vi "holonomic-drive-test.vi"(8 "error in (no error)":errorcluster) -> (0 "error out":errorcluster, 3 "ALL TESTS PASSED":bool)   [LabVIEW 2019]
uses:
  <vilib>/Rock Robotics/WPI/ThirdParty/JAS_Junk/TrajLib/POSE2D.ctl
  <vilib>/Rock Robotics/WPI/ThirdParty/JAS_Junk/TrajLib/TRANSLATION2D.ctl
  <vilib>/Rock Robotics/WPI/ThirdParty/JAS_Junk/TrajLib/ROTATION2D.ctl
  <vilib>/Rock Robotics/WPI/ThirdParty/JAS_Junk/TrajLib/Translation2d_Create.vi
  <vilib>/Rock Robotics/WPI/ThirdParty/JAS_Junk/TrajLib/ProfiledPIDController_NewPeriod.vi
  <vilib>/Rock Robotics/WPI/ThirdParty/JAS_Junk/TrajLib/PIDController_NewPeriod.vi
  <vilib>/Rock Robotics/WPI/ThirdParty/JAS_Junk/TrajLib/ProfiledPIDController_Calculate_Meas_Goal.vi
  <vilib>/Rock Robotics/WPI/ThirdParty/JAS_Junk/TrajLib/ChassisSpeeds_FromFieldRelativeSpeeds.vi
  <vilib>/Rock Robotics/WPI/ThirdParty/JAS_Junk/TrajLib/PIDController_Reset.vi
  <vilib>/Rock Robotics/WPI/ThirdParty/JAS_Junk/TrajLib/PIDController_Calculate_SP_PV.vi
  <vilib>/Rock Robotics/WPI/ThirdParty/JAS_Junk/TrajLib/ProfiledPIDController_Reset_PosOnly.vi
  <vilib>/Rock Robotics/WPI/ThirdParty/JAS_Junk/TrajLib/Rotation2d_GetAngleCosSin.vi
  <vilib>/Rock Robotics/WPI/ThirdParty/JAS_Junk/TrajLib/Pose2d_RelativeTo.vi
  <vilib>/Rock Robotics/WPI/ThirdParty/JAS_Junk/TrajLib/Pose2d_getRotation.vi
  <vilib>/Rock Robotics/WPI/ThirdParty/JAS_Junk/TrajLib/Rotation2d_Minus.vi
  <vilib>/Rock Robotics/WPI/ThirdParty/JAS_Junk/TrajLib/TrapProfState_New.vi
  <vilib>/Rock Robotics/SystemInterfaces/NetworkCommunication/NetComm_UsageReport_report.vi
  <vilib>/Rock Robotics/WPI/ThirdParty/JAS_Junk/TrajLib/ProfiledPIDController_SetGoal_PosOnly.vi
  <vilib>/Rock Robotics/WPI/ThirdParty/JAS_Junk/TrajLib/ProfiledPIDController_Calculate_Meas.vi
  <vilib>/Rock Robotics/WPI/ThirdParty/JAS_Junk/TrajLib/Rotation2d_GetCos.vi
  <vilib>/Rock Robotics/WPI/ThirdParty/JAS_Junk/TrajLib/Rotation2d_GetSin.vi
  <vilib>/Rock Robotics/WPI/ThirdParty/JAS_Junk/TrajLib/ChassisSpeeds_New.vi
  <vilib>/Rock Robotics/WPI/ThirdParty/JAS_Junk/TrajLib/PIDController_SetSetpoint.vi
  <vilib>/Rock Robotics/WPI/ThirdParty/JAS_Junk/TrajLib/PIDController_Calculate_PV.vi
  <vilib>/Rock Robotics/WPI/ThirdParty/JAS_Junk/TrajLib/ProfiledPIDController_Reset.vi
  <vilib>/Rock Robotics/WPI/ThirdParty/JAS_Junk/TrajLib/Transform2d_Create_PosePose.vi
  <vilib>/Rock Robotics/WPI/ThirdParty/JAS_Junk/TrajLib/Pose2d_New_TRRO.vi
  <vilib>/Rock Robotics/WPI/ThirdParty/JAS_Junk/TrajLib/Rotation2d_UnaryMinus.vi
  <vilib>/Rock Robotics/WPI/ThirdParty/JAS_Junk/TrajLib/Rotation2d_RotateBy.vi
  <vilib>/Rock Robotics/WPI/ThirdParty/JAS_Junk/TrajLib/ProfiledPIDController_SetGoal.vi
  <vilib>/Rock Robotics/WPI/ThirdParty/JAS_Junk/TrajLib/TrapProfile_New.vi
  <vilib>/Rock Robotics/WPI/ThirdParty/JAS_Junk/TrajLib/ProfiledPIDController_GetPeriod.vi
  <vilib>/Rock Robotics/WPI/ThirdParty/JAS_Junk/TrajLib/TrapProfile_Calculate.vi
  <vilib>/Rock Robotics/WPI/ThirdParty/JAS_Junk/TrajLib/ControllerUtil_GetModulusError.vi
  <vilib>/Rock Robotics/WPI/ThirdParty/JAS_Junk/TrajLib/Translation2d_RotateBy.vi
  <vilib>/Rock Robotics/WPI/ThirdParty/JAS_Junk/TrajLib/Translation2d_Minus.vi
  <vilib>/Rock Robotics/WPI/ThirdParty/JAS_Junk/TrajLib/Rotation2d_CreateXY.vi
  <vilib>/Rock Robotics/WPI/ThirdParty/JAS_Junk/TrajLib/TrapProfile_ShouldFlipAcceleration.vi
  <vilib>/Rock Robotics/WPI/ThirdParty/JAS_Junk/TrajLib/TrapProfile_Direct.vi
  <vilib>/Rock Robotics/WPI/ThirdParty/JAS_Junk/TrajLib/PIDController_GetPeriod.vi
  <vilib>/Rock Robotics/WPI/ThirdParty/JAS_Junk/TrajLib/Util_CalcDist.vi
  <vilib>/Rock Robotics/WPI/ThirdParty/JAS_Junk/TrajLib/Util_LibraryGlobals.vi
  <vilib>/Rock Robotics/WPI/ThirdParty/JAS_Junk/TrajLib/Trajectory_Library.lvlib
panel:
  out "Test2 Passed":bool
  out "Test2 Omega":dbl
  out "Test2 Y":dbl
  out "Test2 X":dbl
  out "End Angle":dbl
  out "Y Err":dbl
  out "X err":dbl
  out "UpdatedPose":T1 {"ROTATION"."SIN" format="%13.4f"; "ROTATION"."COS" format="%13.4f"; "ROTATION"."VALUE" format="%13.4f"; "TRANSLATION"."Y" format="%14.3f"; "TRANSLATION"."X" format="%14.3f"}
  out "Init Pose":T1 {"ROTATION"."SIN" format="%13.4f"; "ROTATION"."COS" format="%13.4f"; "ROTATION"."VALUE" format="%13.4f"; "TRANSLATION"."Y" format="%14.3f"; "TRANSLATION"."X" format="%14.3f"}
  out "Traj Create Error":errorcluster
  out "Processing Timer Per Pass":dbl
  out "TotalTime":dbl
  out "TotalPasses":dbl
  out "Test Passed":bool
  out "TotalTImeSecs":dbl
  out "Position Graph":cluster{dbl[], dbl[]}[](graph)
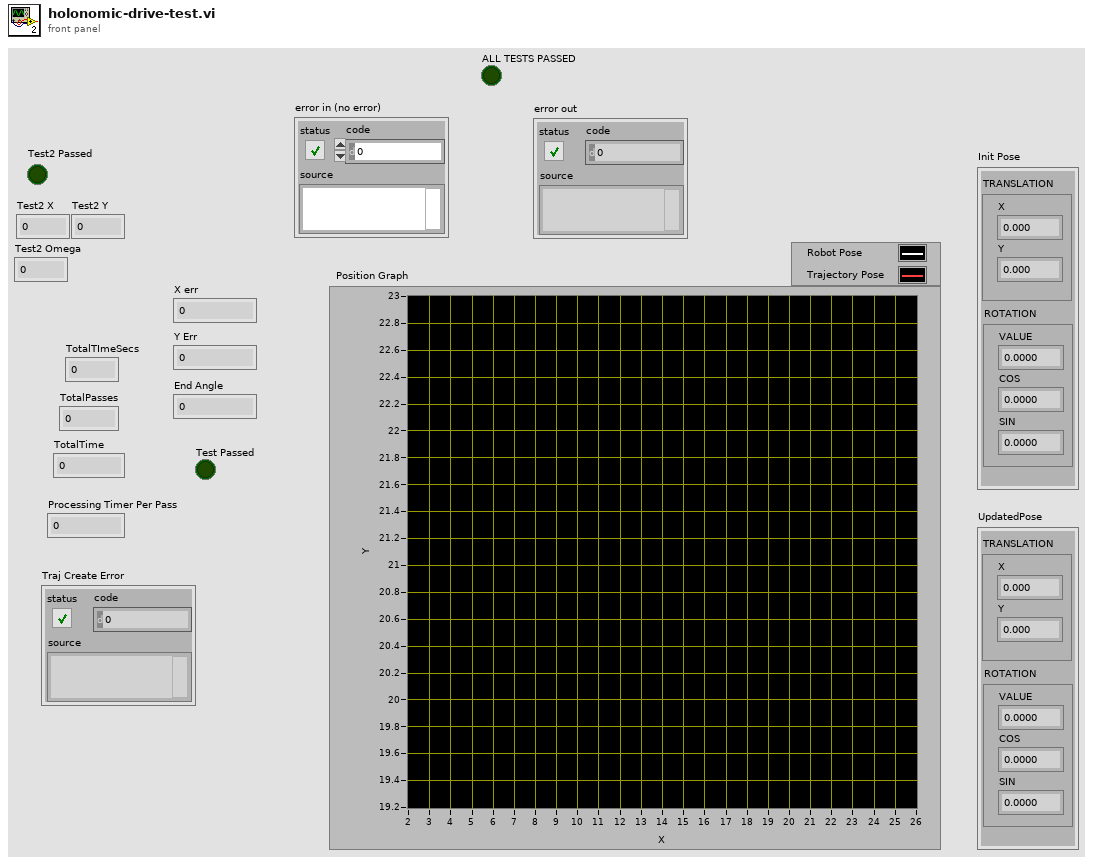
[diagram p1: front panel]
types:
  T1 = typedef "Trajectory_Library.lvlib/POSE2D.ctl" = cluster{"TRANSLATION":T2, "ROTATION":T3}
  T2 = typedef "Trajectory_Library.lvlib/TRANSLATION2D.ctl" = cluster{"X":dbl, "Y":dbl}
  T3 = typedef "Trajectory_Library.lvlib/ROTATION2D.ctl" = cluster{"VALUE":dbl, "COS":dbl, "SIN":dbl}
  T4 = typedef "Trajectory_Library.lvlib/TRAPEZOID_PROFILE_CONSTRAINT.ctl" = cluster{"MaxVelocity":dbl, "MaxAcceleration":dbl}
  T5 = typedef "Trajectory_Library.lvlib/PID_CONTROLLER.ctl" = cluster{"Kp":dbl, "Ki":dbl, "Kd":dbl, "Period":dbl, "Max_Integral":dbl, "Min_Integral":dbl, "Max_Input":dbl, "Min_Input":dbl, "Continuous":bool, "PositionError":dbl, "VelocityError":dbl, "PrevError":dbl, "TotalError":dbl, "PositionTolerance":dbl, "VelocityTolerance":dbl, "SetPoint":dbl, "Kf":dbl, "Prev_Deriv":dbl, "Prev_Deriv 2":dbl, "DerivativeFilter":bool, "Min_Output":dbl, "Max_Output":dbl, "Prev_F_P":dbl, "Prev_F_P_2":dbl, "AntiWindupActive":bool, "Measurement":dbl}
  T6 = typedef "Trajectory_Library.lvlib/PROFILED_PID_CONTROLLER.ctl" = cluster{"Controller":T5, "Goal":T7, "Setpoint":T7, "Constraint":T4}
  T7 = typedef "Trajectory_Library.lvlib/TRAPEZOID_PROFILE_STATE.ctl" = cluster{"Position":dbl, "Velocity":dbl}
  T8 = typedef "Trajectory_Library.lvlib/TRAJ_CONFIG.ctl" = cluster{"MaxVelocity":dbl, "Max Acceleration":dbl, "StartVelocity":dbl, "End Velocity":dbl, "Reversed":bool, "DiffDrKineConstntDefined":bool, "CentAcellConstntDefined":bool, "DiffDrVoltConstntDefined":bool, "DIFF_DRIVE_KINE_CONSTRAINT":T9, "CENTRIPETAL_ACCEL_CONSTRAINT":T11, "SwerveDrKineConstntDefined":bool, "SWERVE_DRIVE_KINE_CONSTRAINT":T12, "DIFF_DRIVE_VOLTAGE_CONSTRAINT":T15, "MECANUM_DRIVE_KINE_CONSTRAINT":T17, "MecanumDrKineConstntDefined":bool}
  T9 = typedef "Trajectory_Library.lvlib/TRAJ_CONSTRAINT_DIIF_DRIVE_KINEMATICS.ctl" = cluster{"Max Speed (M/S)":dbl, "DIFF_DRIVE_KINEMATICS":T10, "Max Accel (M/S2)":dbl}
  T10 = typedef "Trajectory_Library.lvlib/DIFF_DRIVE_KINEMATICS.ctl" = cluster{"TrackWidth_Meters":dbl}
  T11 = typedef "Trajectory_Library.lvlib/TRAJ_CONSTRAINT_CENTRIPETAL_ACCEL.ctl" = cluster{"Max Cent Accel":dbl}
  T12 = typedef "Trajectory_Library.lvlib/TRAJ_CONSTRAINT_SWERVE_DRIVE_KINEMATICS.ctl" = cluster{"Max Speed (M/S)":dbl, "SwerveKinematics":T13}
  T13 = typedef "Trajectory_Library.lvlib/SWERVE_DRIVE_KINEMATICS.ctl" = cluster{"NumModules":i32, "InverseKinematics":T14, "ForwardKinematics":T14, "Modules":T2[], "PrevCoR":T2}
  T14 = typedef "NI_Matrix.lvlib/RealMatrix.ctl" = dbl[][]
  T15 = typedef "Trajectory_Library.lvlib/TRAJ_CONSTRAINT_DIIF_DRIVE_VOLTAGE.ctl" = cluster{"Max Voltage":dbl, "DIFF_DRIVE_KINEMATICS":T10, "SIMPLE_MOTOR_FF":T16}
  T16 = typedef "Trajectory_Library.lvlib/SIMPLE_MOTOR_FF.ctl" = cluster{"Ks":dbl, "Kv":dbl, "Ka":dbl}
  T17 = typedef "Trajectory_Library.lvlib/TRAJ_CONSTRAINT_MECA_DRIVE_KINEMATICS.ctl" = cluster{"Max Speed (M/S)":dbl, "MECA_DRIVE_KINEMATICS":T18}
  T18 = typedef "Trajectory_Library.lvlib/MECA_DRIVE_KINEMATICS.ctl" = cluster{"FrontLeft":T2, "FrontRight":T2, "RearLeft":T2, "RearRight":T2, "InverseKinematics":T14, "ForwardKinematics":T14, "PrevCoR":T2}
  T19 = typedef "Trajectory_Library.lvlib/HOLONOMIC_DRV_CTRL.ctl" = cluster{"poseTolerance":T1, "poseError":T1, "Enabled":bool, "PID_xCtrl":T5, "PID_yCtrl":T5, "PROF_PID_thetaCtrl":T6, "RotationError":T3, "FirstRun":bool}
  T20 = typedef "Trajectory_Library.lvlib/TRAJECTORY.ctl" = cluster{"TotalTImeSecs":dbl, "States":T21[]}
  T21 = typedef "Trajectory_Library.lvlib/TRAJ_STATE.ctl" = cluster{"TimeSeconds":dbl, "Velocity":dbl, "Acceleration":dbl, "POSE":T1, "Curvature":dbl}
  T22 = typedef "Trajectory_Library.lvlib/CHASSIS_SPEEDS.ctl" = cluster{"vX":dbl, "vY":dbl, "vOmega":dbl}
  T23 = typedef "Trajectory_Library.lvlib/TWIST2D.ctl" = cluster{"dX":dbl, "dY":dbl, "dTHETA":dbl}
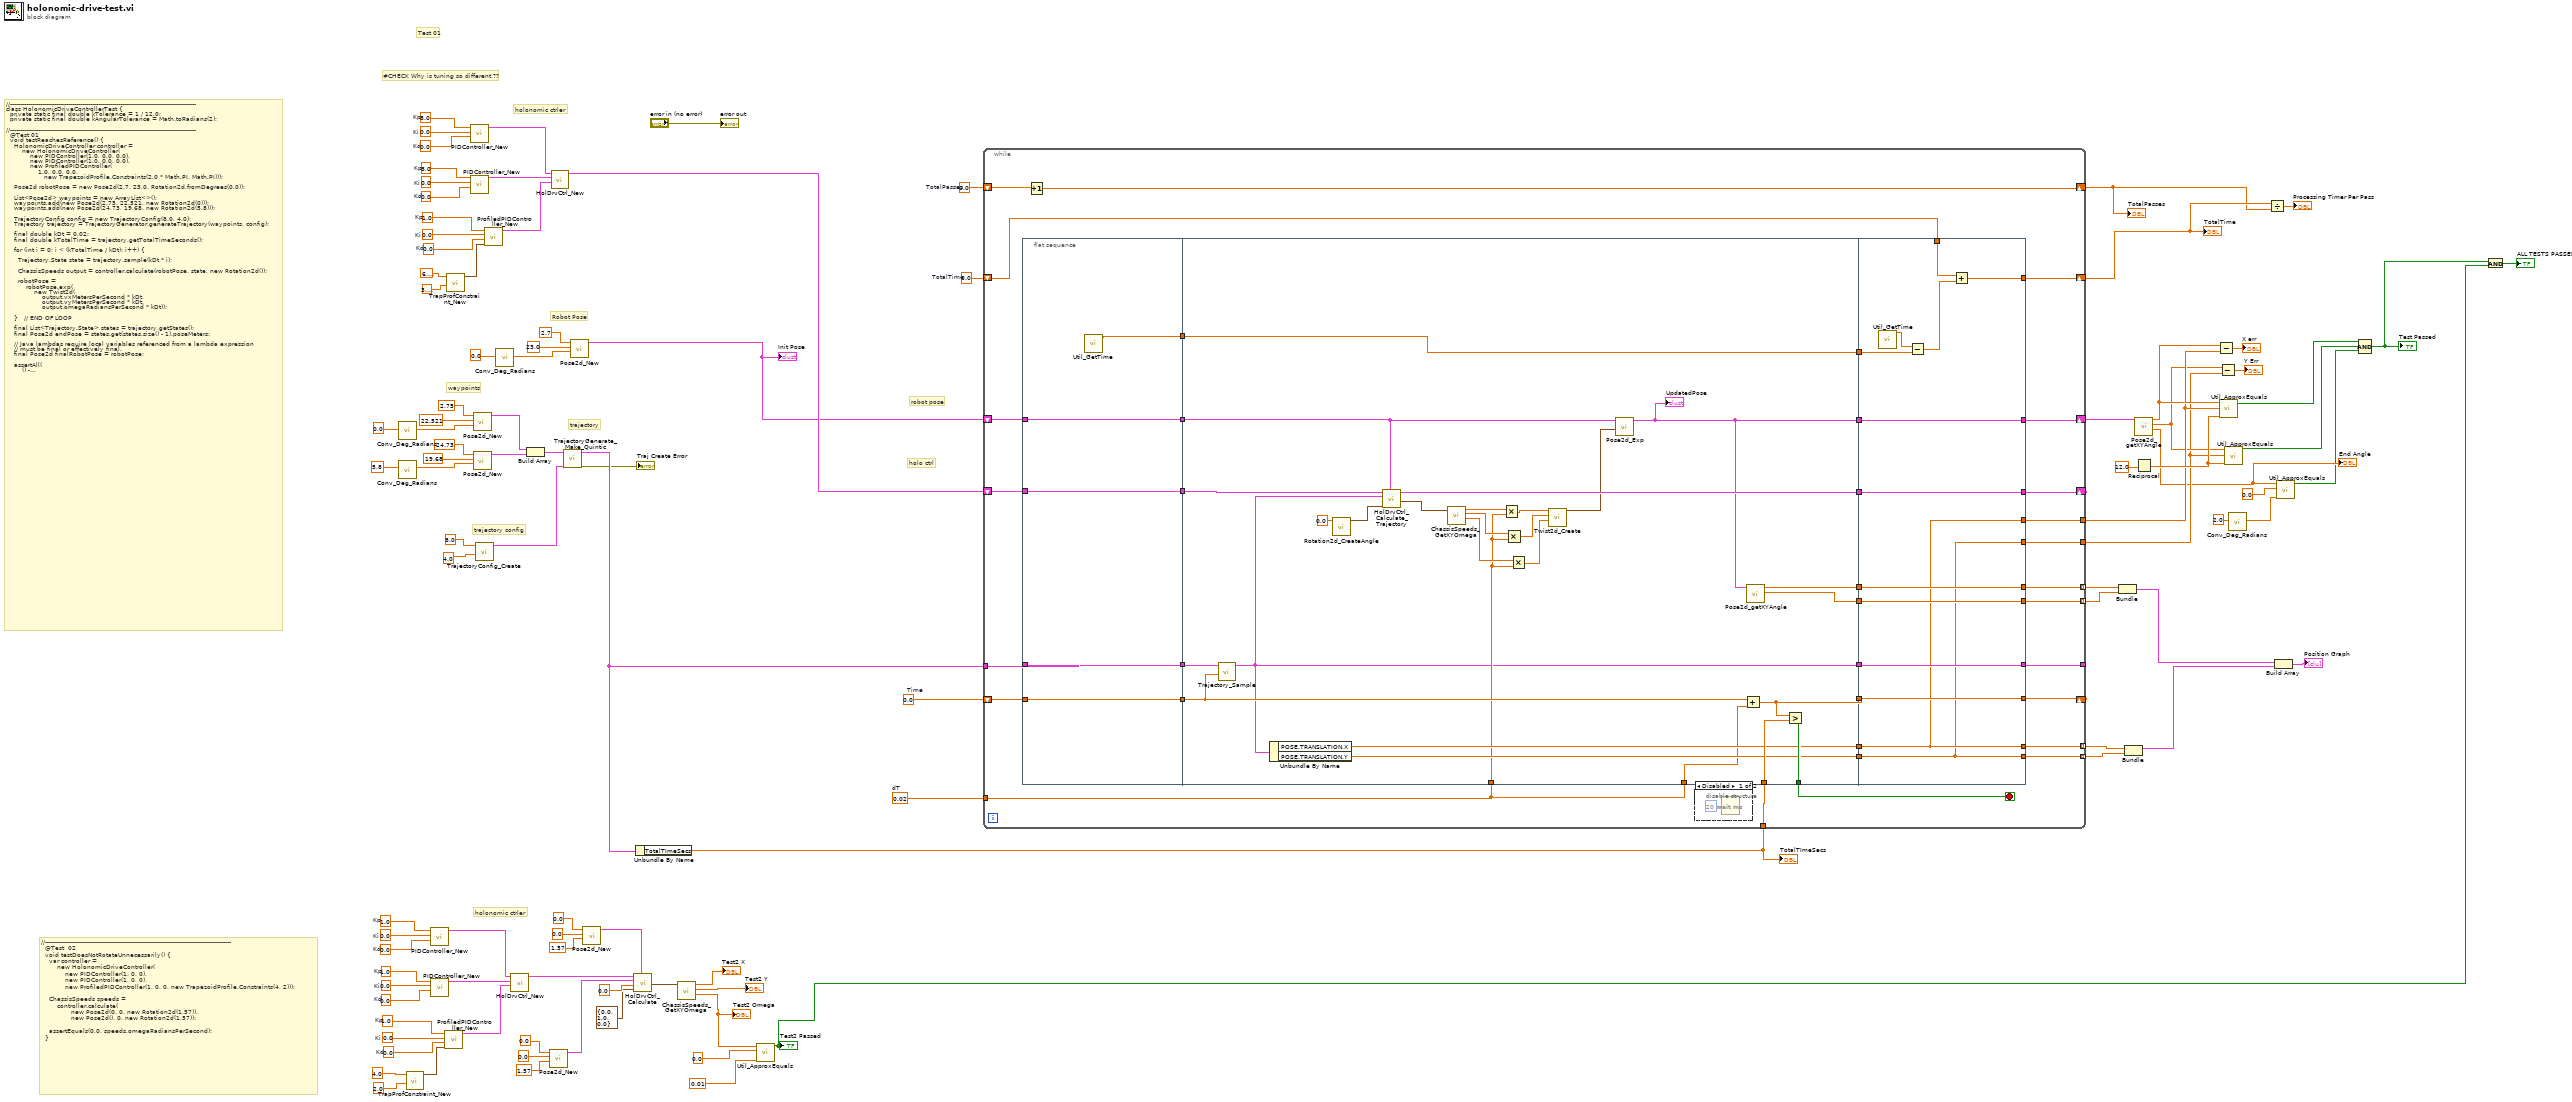
[diagram p0: block diagram]
diagram:
  w23 = 1.0  # Kp
  w24 = 0.0  # Ki
  w25 = 0.0  # Kd
  w29 = 1.0  # Kp
  w30 = 0.0  # Ki
  w31 = 0.0  # Kd
  w32 = 1.0  # Kp
  w33 = 0.0  # Ki
  w34 = 0.0  # Kd
  w56 = 0.02  # dT
  w65 = 1.0  # Kp
  w66 = 0.0  # Ki
  w67 = 0.0  # Kd
  w71 = 8.0  # Kp
  w72 = 0.0  # Ki
  w73 = 0.0  # Kd
  w74 = 8.0  # Kp
  w75 = 0.0  # Ki
  w76 = 0.0  # Kd
  w80 = 0.0  # TotalPasses
  w81 = 0.0  # TotalTime
  w90 = 0.0  # Time
  # "holonomic ctrler"
  # "//---------------------------------------------------------------------------------------------\n  @Test  02\n  void testDoesNotRotateUnnecessarily() {\n    var controller =\n        new HolonomicDriveController(\n            new PIDController(1, 0, 0),\n            new PIDController(1, 0, 0),\n            new ProfiledPIDController(1, 0, 0, new TrapezoidProfile.Constraints(4, 2)));\n\n    ChassisSpeeds speeds =\n        controller.calculate(\n               new Pose2d(0, 0, new Rotation2d(1.57)), \n               new Pose2d(), 0, new Rotation2d(1.57));\n\n    assertEquals(0.0, speeds.omegaRadiansPerSecond);\n  }"
  # "#CHECK Why is tuning so different ??"
  # "robot pose"
  # "holo ctrl"
  # "holonomic ctrler"
  # "Test 01"
  # "Robot Pose"
  # "//---------------------------------------------------------------------------------------------\nclass HolonomicDriveControllerTest {\n  private static final double kTolerance = 1 / 12.0;\n  private static final double kAngularTolerance = Math.toRadians(2);\n\n//---------------------------------------------------------------------------------------------\n  @Test 01\n  void testReachesReference() {\n    HolonomicDriveController controller =\n        new HolonomicDriveController(\n            new PIDController(1.0, 0.0, 0.0),\n            new PIDController(1.0, 0.0, 0.0),\n            new ProfiledPIDController(\n                1.0, 0.0, 0.0, \n                   new TrapezoidProfile.Constraints(2.0 * Math.PI, Math.PI)));\n\n    Pose2d robotPose = new Pose2d(2.7, 23.0, Rotation2d.fromDegrees(0.0));\n\n    List<Pose2d> waypoints = new ArrayList<>();\n    waypoints.add(new Pose2d(2.75, 22.521, new Rotation2d(0)));\n    waypoints.add(new Pose2d(24.73, 19.68, new Rotation2d(5.8)));\n\n    TrajectoryConfig config = new TrajectoryConfig(8.0, 4.0);\n    Trajectory trajectory = TrajectoryGenerator.generateTrajectory(waypoints, config);\n\n    final double kDt = 0.02;\n    final double kTotalTime = trajectory.getTotalTimeSeconds();\n\n    for (int i = 0; i < (kTotalTime / kDt); i++) {\n\n      Trajectory.State state = trajectory.sample(kDt * i);\n\n      ChassisSpeeds output = controller.calculate(robotPose, state, new Rotation2d());\n\n      robotPose =\n          robotPose.exp(\n              new Twist2d(\n                  output.vxMetersPerSecond * kDt,\n                  output.vyMetersPerSecond * kDt,\n                  output.omegaRadiansPerSecond * kDt));\n\n    }   // END OF LOOP\n\n    final List<Trajectory.State> states = trajectory.getStates();\n    final Pose2d endPose = states.get(states.size() - 1).poseMeters;\n\n    // Java lambdas require local variables referenced from a lambda expression\n    // must be final or effectively final.\n    final Pose2d finalRobotPose = robotPose;\n\n    assertAll(\n        () -> assertEquals(endPose.getX(), finalRobotPose.getX(), kTolerance),\n        () -> assertEquals(endPose.getY(), finalRobotPose.getY(), kTolerance),\n        () ->\n            assertEquals(\n                0.0,\n                MathUtil.angleModulus(finalRobotPose.getRotation().getRadians()),\n                kAngularTolerance));\n  }\n}"
  # "trajectory config"
  # "trajectory"
  # "waypoints"
  n1 = call <vilib>:"Conv_Deg_Radians.vi"("Degress"=0.0 ("Heading")) -> ("Radians"=w94:dbl)  [unwired: 10 in]
  n2 = call <vilib>:"Conv_Deg_Radians.vi"("Degress"=5.8 ("Heading")) -> ("Radians"=w98:dbl)  [unwired: 10 in]
  n3 = call <vilib>:"TrapProfConstraint_New.vi"("Max Accel"=2.0, "Max Speed (M/S)"=4.0) -> ("TRAPEZOID_PROFILE_CONSTRAINT"=w26:T4)  [unwired: 9 in]
  n4 = call <vilib>:"PIDController_New.vi"("Kd"=w34, "Ki"=w33, "Kp"=w32) -> ("PID_CONTROLLER"=w28:T5)  [unwired: 8 in]
  n5 = call <vilib>:"PIDController_New.vi"("Kd"=w31, "Ki"=w30, "Kp"=w29) -> ("PID_CONTROLLER"=w27:T5)  [unwired: 8 in]
  n6 = call <vilib>:"ProfiledPIDController_New.vi"("Constraints"=w26, "Kd"=w25, "Ki"=w24, "Kp"=w23) -> ("PROFILED_PID_CONTROLLER"=w22:T6)  [unwired: 7 in]
  n7 = call <vilib>:"TrapProfConstraint_New.vi"("Max Accel"=3.141592653589793, "Max Speed (M/S)"=6.283185307179586) -> ("TRAPEZOID_PROFILE_CONSTRAINT"=w68:T4)  [unwired: 9 in]
  n8 = call <vilib>:"PIDController_New.vi"("Kd"=w76, "Ki"=w75, "Kp"=w74) -> ("PID_CONTROLLER"=w70:T5)  [unwired: 8 in]
  n9 = call <vilib>:"PIDController_New.vi"("Kd"=w73, "Ki"=w72, "Kp"=w71) -> ("PID_CONTROLLER"=w69:T5)  [unwired: 8 in]
  n10 = call <vilib>:"Pose2d_New.vi"("Heading"=w94, "Y"=22.521, "X"=2.75) -> ("out POSe"=w93:T1)  [unwired: 8 in]
  n11 = call <vilib>:"Pose2d_New.vi"("Heading"=w98, "Y"=19.68, "X"=24.73) -> ("out POSe"=w91:T1)  [unwired: 8 in]
  n12 = call <vilib>:"TrajectoryConfig_Create.vi"("MaxAcceleration"=4.0, "MaxVelocity"=8.0) -> ("TRAJECTORY_CONFIG"=w102:T8)  [unwired: 9 in]
  n13 = call <vilib>:"ProfiledPIDController_New.vi"("Constraints"=w68, "Kd"=w67, "Ki"=w66, "Kp"=w65) -> ("PROFILED_PID_CONTROLLER"=w64:T6)  [unwired: 7 in]
  n14 = call <vilib>:"Conv_Deg_Radians.vi"("Degress"=0.0 ("Heading")) -> ("Radians"=w58:dbl)  [unwired: 10 in]
  n15 = call <vilib>:"HolDrvCtrl_New.vi"("thetaProfiledPID_CTRL"=w22, "yPID_CTRL"=w27, "xPID_CTRL"=w28) -> ("outHOLONOMIC_DRV_CTRL"=w19:T19)  [unwired: 8 in]
  n16 = Build Array(w93, w91) -> (w103:T1[])
  n17 = call <vilib>:"Pose2d_New.vi"("Heading"=1.57, "Y"=0.0, "X"=0.0) -> ("out POSe"=w12:T1)  [unwired: 8 in]
  n18 = call <vilib>:"HolDrvCtrl_New.vi"("thetaProfiledPID_CTRL"=w64, "yPID_CTRL"=w69, "xPID_CTRL"=w70) -> ("outHOLONOMIC_DRV_CTRL"=w55:T19)  [unwired: 8 in]
  n19 = call <vilib>:"TrajectoryGenerate_Make_Quintic.vi"("traj_config"=w102, "waypointPOSE"=w103) -> ("error out"=→"Traj Create Error":errorcluster, "TRAJECTORY"=w89:T20)  [unwired: 8 in]
  n20 = call <vilib>:"Pose2d_New.vi"("Heading"=w58, "Y"=23.0, "X"=2.7) -> ("out POSe"=w54:T1)  [unwired: 8 in]
  "Init Pose" <- w54
  n21 = call <vilib>:"Pose2d_New.vi"("Heading"=1.57, "Y"=0.0, "X"=0.0) -> ("out POSe"=w11:T1)  [unwired: 8 in]
  n22 = call <vilib>:"HolDrvCtrl_Calculate.vi"("currentPose"=w11, "angleRef"=T3 {"VALUE"=0.0, "COS"=1.0, "SIN"=0.0}, "linearVelRef"=0.0, "poseRef"=w12, "inHOLONOMIC_DRV_CTRL"=w19) -> ("calcChassisSpeed"=w8:T22)  [unwired: 5 in, 1 out]
  n23 = Unbundle By Name(w89) -> ("TotalTImeSecs"=w82:dbl)
  "TotalTImeSecs" <- w82
  n24 = call <vilib>:"ChassisSpeeds_GetXYOmega.vi"("CHASSIS"=w8) -> ("vAngular"=w5:dbl, "vY"=→"Test2 Y":dbl, "vX"=→"Test2 X":dbl)  [unwired: 8 in]
  "Test2 Omega" <- w5
  n25 = call <vilib>:"Util_ApproxEquals.vi"("Tolerance"=0.01, "Value 2"=0.0, "Value 1"=w5) -> ("ApproxEquals"=w3:bool)  [unwired: 8 in]
  "Test2 Passed" <- w3
  n26 = while {
    shift-right: [w139] -> _
    shift-left: w90 -> [w136]
    tunnel: w89 -> [w137]
    tunnel: w82 -> [w138]
    tunnel: [w135] -> w88 mode=indexing
    tunnel: [w134] -> w87 mode=indexing
    tunnel: [w133] -> w85 mode=indexing
    tunnel: [w132] -> w84 mode=indexing
    shift-right: [w121] -> w79
    shift-left: w81 -> [w120]
    shift-right: [w118] -> w78
    shift-left: w80 -> [w119]
    tunnel: w56 -> [w111]
    shift-right: [w113] -> _
    shift-left: w55 -> [w117]
    shift-right: [w110] -> w52
    shift-left: w54 -> [w114]
    tunnel: [w108] -> _
    tunnel: [w106] -> w48
    tunnel: [w105] -> w46
    stop <- w131 stop-if-true
    n27 = flat-sequence {
      tunnel: w136 -> [w144]
      tunnel: w137 -> [w145]
      tunnel: [w145] -> w130
      tunnel: [w144] -> w129
      tunnel: [w143] -> w123
      tunnel: w117 -> [w142]
      tunnel: [w142] -> w116
      tunnel: [w141] -> w115
      tunnel: w114 -> [w141]
      tunnel: [w172] -> w131
      tunnel: w138 -> [w170]
      tunnel: w130 -> [w169]
      tunnel: w129 -> [w168]
      tunnel: [w171] -> w128
      tunnel: [w151] -> w127
      tunnel: [w150] -> w126
      tunnel: [w167] -> w125
      tunnel: [w166] -> w124
      tunnel: w123 -> [w165]
      tunnel: [w165] -> w122
      tunnel: w111 -> [w164]
      tunnel: w116 -> [w163]
      tunnel: w115 -> [w161]
      tunnel: [w162] -> w112
      tunnel: w111 -> [w156]
      tunnel: [w149] -> w109
      tunnel: [w148] -> w107
      tunnel: [w174] -> w132
      tunnel: [w173] -> w133
      tunnel: [w183] -> w134
      tunnel: [w184] -> w135
      tunnel: [w185] -> w139
      tunnel: w128 -> [w185]
      tunnel: w127 -> [w184]
      tunnel: w126 -> [w183]
      tunnel: w125 -> [w173]
      tunnel: w124 -> [w174]
      tunnel: w122 -> [w181]
      tunnel: [w180] -> w121
      tunnel: w120 -> [w178]
      tunnel: [w177] -> w113
      tunnel: w112 -> [w177]
      tunnel: [w176] -> w110
      tunnel: w109 -> [w176]
      tunnel: [w175] -> w108
      tunnel: w107 -> [w175]
      tunnel: [w174] -> w106
      tunnel: [w173] -> w105
      frame #0 {
        n28 = call <vilib>:"Util_GetTime.vi"() -> ("FPGA_Time_Seconds"=w143:dbl)  [unwired: 10 in, 1 out]
      }
      frame #1 {
        n29 = call <vilib>:"Trajectory_Sample.vi"("Time"=w168, "InputTRAJECTORY"=w169) -> ("OutputTRAJ_STATE"=w148:T21)  [unwired: 9 in]
        n30 = Unbundle By Name(w148) -> ("POSE.TRANSLATION.X"=w166:dbl, "POSE.TRANSLATION.Y"=w167:dbl)
        n31 = call <vilib>:"Rotation2d_CreateAngle.vi"("Angle"=0.0) -> ("ROTATION"=w146:T3)  [unwired: 10 in]
        n32 = call <vilib>:"HolDrvCtrl_Calculate_Trajectory.vi"("currentPose"=w161, "angleRef"=w146, "desiredTrajState"=w148, "inHOLONOMIC_DRV_CTRL"=w163) -> ("calcChassisSpeed"=w160:T22, "outHOLONOMIC_DRV_CTRL"=w162:T19)  [unwired: 6 in]
        n33 = call <vilib>:"ChassisSpeeds_GetXYOmega.vi"("CHASSIS"=w160) -> ("vAngular"=w157:dbl, "vY"=w158:dbl, "vX"=w159:dbl)  [unwired: 8 in]
        n34 = Multiply(x=w159, y=w156) -> (x*y=w155:dbl)
        n35 = Multiply(x=w158, y=w156) -> (x*y=w154:dbl)
        n36 = Multiply(x=w157, y=w156) -> (x*y=w153:dbl)
        n37 = call <vilib>:"Twist2d_Create.vi"("dTHETA"=w153, "dY"=w154, "dX"=w155) -> ("TWIST"=w152:T23)  [unwired: 8 in]
        n38 = call <vilib>:"Pose2d_Exp.vi"("TWIST"=w152, "POSE"=w161) -> ("UpdatedPose"=w149:T1)  [unwired: 9 in]
        "UpdatedPose" <- w149
        n39 = Add(x=w168, y=w164) -> (x+y=w171:dbl)
        n40 = call <vilib>:"Pose2d_getXYAngle.vi"("in POSE"=w149) -> ("Y"=w150:dbl, "X"=w151:dbl)  [unwired: 8 in, 1 out]
        n41 = Greater?(x=w171, y=w170) -> (0:w172:bool)
      }
      frame #2 {
        n42 = call <vilib>:"Util_GetTime.vi"() -> ("FPGA_Time_Seconds"=w182:dbl)  [unwired: 10 in, 1 out]
        n43 = Subtract(x=w182, y=w181) -> (x-y=w179:dbl)
        n44 = Add(x=w178, y=w179) -> (x+y=w180:dbl)
      }
    }
    n45 = Increment(x=w119) -> (x+1=w118:dbl)
    n46 = disable-structure shown="Disabled" {
      frame Disabled {
        n47 = Wait (ms)(milliseconds to wait=u32 20) -> ()  [unwired: 1 out]
      }
      frame Enabled {
      }
    }
  }
  "TotalPasses" <- w78
  "TotalTime" <- w79
  n48 = Bundle(w88, w87) -> (w53:cluster{dbl[], dbl[]})  [unwired: 1 in]
  n49 = Bundle(w84, w85) -> (w83:cluster{dbl[], dbl[]})  [unwired: 1 in]
  n50 = call <vilib>:"Pose2d_getXYAngle.vi"("in POSE"=w52) -> ("Angle"=w41:dbl, "Y"=w47:dbl, "X"=w49:dbl)  [unwired: 8 in]
  "End Angle" <- w41
  n51 = Reciprocal(x=12.0) -> (1/x=w50:dbl)
  n52 = Subtract(x=w49, y=w48) -> (x-y=→"X err":dbl)
  n53 = Subtract(x=w47, y=w46) -> (x-y=→"Y Err":dbl)
  n54 = call <vilib>:"Util_ApproxEquals.vi"("Tolerance"=w50, "Value 2"=w48, "Value 1"=w49) -> ("ApproxEquals"=w43:bool)  [unwired: 8 in]
  n55 = call <vilib>:"Util_ApproxEquals.vi"("Tolerance"=w50, "Value 2"=w46, "Value 1"=w47) -> ("ApproxEquals"=w42:bool)  [unwired: 8 in]
  n56 = call <vilib>:"Conv_Deg_Radians.vi"("Degress"=2.0) -> ("Radians"=w38:dbl)  [unwired: 10 in]
  n57 = Divide(x=w79, y=w78) -> (x/y=→"Processing Timer Per Pass":dbl)
  n58 = Build Array(w53, w83) -> (→"Position Graph":cluster{dbl[], dbl[]}[])
  n59 = call <vilib>:"Util_ApproxEquals.vi"("Tolerance"=w38, "Value 2"=0.0, "Value 1"=w41) -> ("ApproxEquals"=w37:bool)  [unwired: 8 in]
  n60 = Compound Arithmetic op=AND(w43, w42, w37) -> (w35:bool)
  "Test Passed" <- w35
  n61 = And(x=w35, y=w3) -> (x .and. y?=→"ALL TESTS PASSED":bool)
  "error out" <- "error in (no error)"
